vi "Get Names.vi"(8 "error in (no error)":errorcluster, 11 "Orange Plugin in":refnum<class "Orange Plugin.lvclass">) -> (0 "error out":errorcluster, 2 "Name":string, 3 "Orange Plugin out":refnum<class "Orange Plugin.lvclass">)   [LabVIEW 2020, in "Orange Plugin.lvclass"]
uses:
  Orange Plugin.lvclass
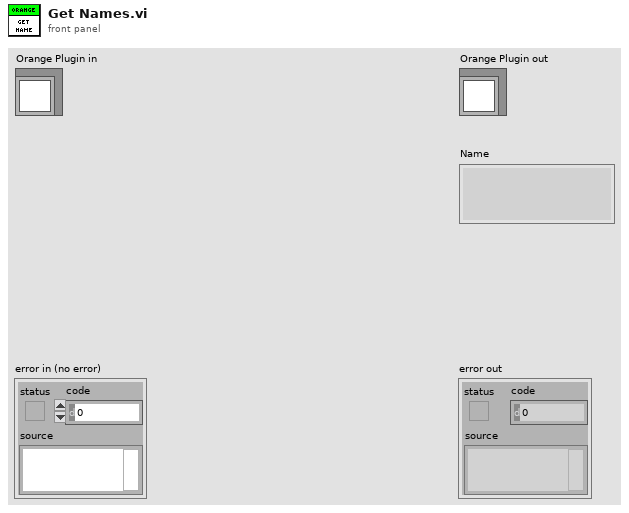
[diagram p1: front panel]
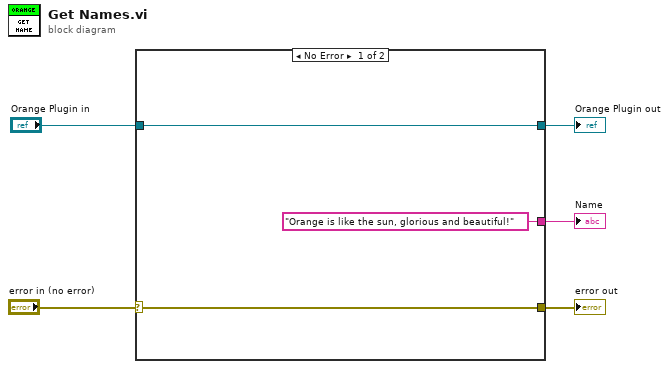
[diagram p0: block diagram]
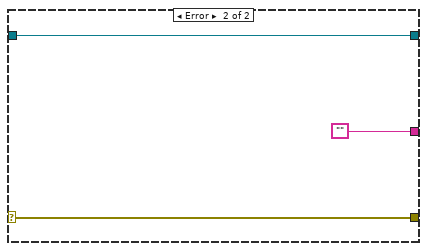
[diagram p2: hidden frame]
diagram:
  n1 = case shown="No Error" "error in (no error)" {
    selector: "error in (no error)" -> [w8 w11]
    tunnel: [w8 w11] -> w4
    tunnel: "Orange Plugin in" -> [w7 w10]
    tunnel: [w7 w10] -> w2
    tunnel: ["Orange is like the sun, glorious and beautiful!" ""] -> w1
    frame No Error {
    }
    frame Error {
    }
  }
  "error out" <- w4
  "Orange Plugin out" <- w2
  "Name" <- w1
